vi "Log Write.vi"(6 "Controller Data In":refnum<data-value>, 7 "Write Header":bool, 8 "Measurement In":refnum<data-value>, 9 "State Estimate In":refnum<data-value>, 10 "Log Handle In":T1, 11 "Error In":errorcluster) -> (0 "Measurement Out":refnum<data-value>, 1 "State Estimate Out":refnum<data-value>, 2 "Log Handle Out":T1, 3 "Error Out":errorcluster, 4 "Controller Data Out":refnum<data-value>, 5 "Logged Events":string[](array[string]))   [LabVIEW 2021]
uses:
  State Estimator/Measurements.ctl
  IMU/IMU Data.ctl
  Steering Motor Encoder/Steering Motor Encoder Data.ctl
  GNSS/GNSS Data.ctl
  State Estimator/State Estimate.ctl
  Log Handle.ctl
  Controller Data.ctl
  Drive Motor/Drive Motor Data.ctl
  Steering Motor/Steering Motor Data.ctl
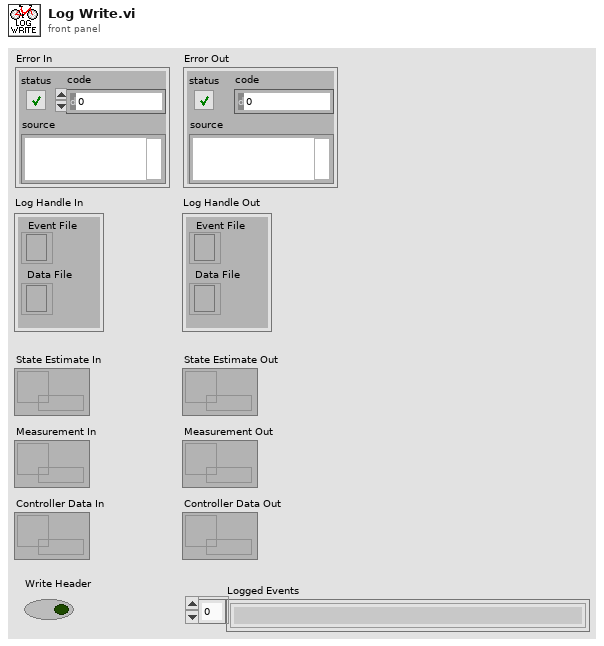
[diagram p1: front panel]
types:
  T1 = typedef "Log Handle.ctl" = cluster{"Data File":refnum<file>, "Event File":refnum<file>}
  T2 = typedef "State Estimate.ctl" = cluster{"X (m)":dbl, "Y (m)":dbl, "Psi (rad)":dbl, "Roll (rad)":dbl, "Roll Rate (rad/s)":dbl}
  T3 = typedef "Controller Data.ctl" = cluster{"Drive Motor Data":T4, "Steering Motor Data":T5}
  T4 = typedef "Drive Motor Data.ctl" = cluster{"Angular Speed (rad/s)":dbl, "Input Current (A)":dbl, "Motor Current (A)":dbl, "MOSFET Temperature (deg C)":dbl}
  T5 = typedef "Steering Motor Data.ctl" = cluster{"PWM":dbl, "Steering Angle Rate (rad/s)":dbl}
  T6 = typedef "Measurements.ctl" = cluster{"IMU Data":T7, "Steering Motor Encoder Data":T8, "GNSS Data":T9}
  T7 = typedef "IMU Data.ctl" = cluster{"Gyroscope":cluster{"X (rad/s)":dbl, "Y (rad/s)":dbl, "Z (rad/s)":dbl}, "Accelerometer":cluster{"X (m/s^2)":dbl, "Y (m/s^2)":dbl, "Z (m/s^2)":dbl}}
  T8 = typedef "Steering Motor Encoder Data.ctl" = cluster{"Encoder Position (counts)":i32, "Steering Angle (rad)":dbl}
  T9 = typedef "GNSS Data.ctl" = cluster{"Latitude (rad)":dbl, "Longitude (rad)":dbl, "Altitude (m)":dbl, "Speed (m/s)":dbl, "Heading (rad)":dbl, "Fix Quality":i32, "Number of Satellites":i32, "Latitude (deg)":dbl, "Longitude (deg)":dbl}
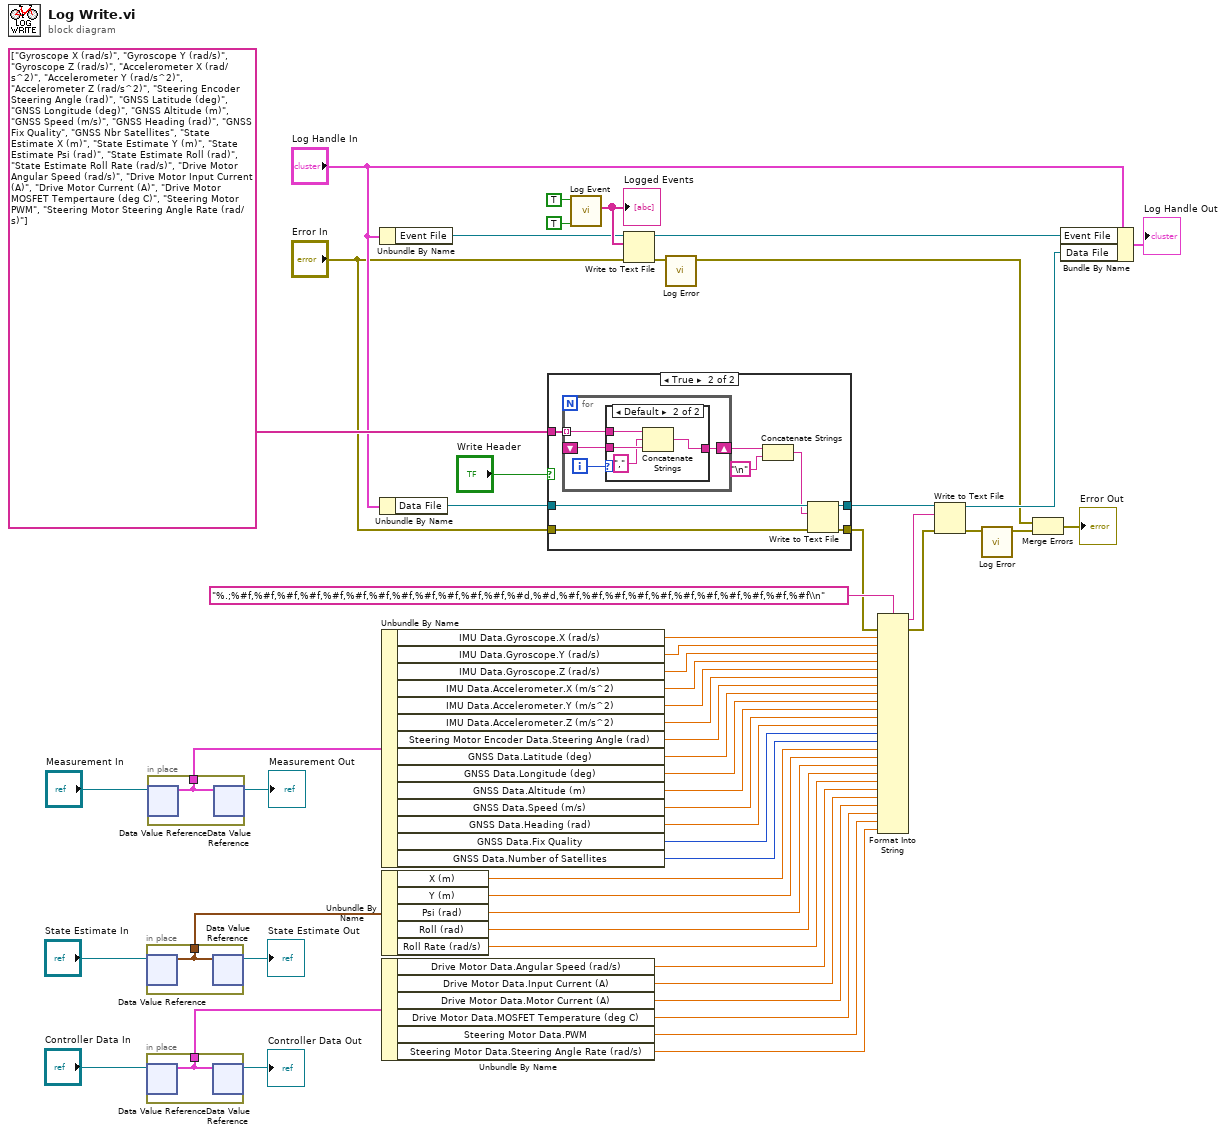
[diagram p0: block diagram]
diagram:
  n1 = in-place {
    in-place-border: [w57] -> w51
    n2 = in-place-dvr #1("State Estimate In") -> (w57:T2)  [unwired: 1 out]
    n3 = in-place-dvr #1(w57) -> (→"State Estimate Out":refnum<data-value>)  [unwired: 1 out]
  }
  n4 = in-place {
    in-place-border: [w58] -> w7
    n5 = in-place-dvr #2("Controller Data In") -> (w58:T3)  [unwired: 1 out]
    n6 = in-place-dvr #2(w58) -> (→"Controller Data Out":refnum<data-value>)  [unwired: 1 out]
  }
  n7 = in-place {
    in-place-border: [w59] -> w52
    n8 = in-place-dvr #3("Measurement In") -> (w59:T6)  [unwired: 1 out]
    n9 = in-place-dvr #3(w59) -> (→"Measurement Out":refnum<data-value>)  [unwired: 1 out]
  }
  n10 = Unbundle By Name("Log Handle In") -> ("Event File"=w19:refnum<file>)
  n11 = Unbundle By Name("Log Handle In") -> ("Data File"=w49:refnum<file>)
  n12 = Unbundle By Name(w52) -> ("IMU Data.Gyroscope.X (rad/s)"=w47:dbl, "IMU Data.Gyroscope.Y (rad/s)"=w46:dbl, "IMU Data.Gyroscope.Z (rad/s)"=w45:dbl, "IMU Data.Accelerometer.X (m/s^2)"=w44:dbl, "IMU Data.Accelerometer.Y (m/s^2)"=w43:dbl, "IMU Data.Accelerometer.Z (m/s^2)"=w42:dbl, "Steering Motor Encoder Data.Steering Angle (rad)"=w41:dbl, "GNSS Data.Latitude (deg)"=w40:dbl, "GNSS Data.Longitude (deg)"=w39:dbl, "GNSS Data.Altitude (m)"=w38:dbl, "GNSS Data.Speed (m/s)"=w37:dbl, "GNSS Data.Heading (rad)"=w36:dbl, "GNSS Data.Fix Quality"=w35:i32, "GNSS Data.Number of Satellites"=w34:i32)
  n13 = Unbundle By Name(w51) -> ("X (m)"=w32:dbl, "Y (m)"=w31:dbl, "Psi (rad)"=w30:dbl, "Roll (rad)"=w29:dbl, "Roll Rate (rad/s)"=w28:dbl)
  n14 = Unbundle By Name(w7) -> ("Drive Motor Data.Angular Speed (rad/s)"=w6:dbl, "Drive Motor Data.Input Current (A)"=w5:dbl, "Drive Motor Data.Motor Current (A)"=w4:dbl, "Drive Motor Data.MOSFET Temperature (deg C)"=w3:dbl, "Steering Motor Data.PWM"=w2:dbl, "Steering Motor Data.Steering Angle Rate (rad/s)"=w1:dbl)
  n15 = case shown="True" "Write Header" {
    tunnel: string[] ["Gyroscope X (rad/s)", "Gyroscope Y (rad/s)", "Gyroscope Z (rad/s)", "Accelerometer X (rad/s^2)", "Accelerometer Y (rad/s^2)", "Accelerometer Z (rad/s^2)", "Steering Encoder Steering Angle (rad)", "GNSS Latitude (deg)", "GNSS Longitude (deg)", "GNSS Altitude (m)", "GNSS Speed (m/s)", "GNSS Heading (rad)", "GNSS Fix Quality", "GNSS Nbr Satellites", "State Estimate X (m)", "State Estimate Y (m)", "State Estimate Psi (rad)", "State Estimate Roll (rad)", "State Estimate Roll Rate (rad/s)", "Drive Motor Angular Speed (rad/s)", "Drive Motor Input Current (A)", "Drive Motor Current (A)", "Drive Motor MOSFET Tempertaure (deg C)", "Steering Motor PWM", "Steering Motor Steering Angle Rate (rad/s)"] ("channel name(s) in (Untitled)") -> [_ w69]
    tunnel: w49 -> [w61 w68]
    tunnel: "Error In" -> [w60 w67]
    tunnel: [w61 w66] -> w27
    tunnel: [w60 w65] -> w25
    frame False {
    }
    frame True {
      n16 = for {
        tunnel: w69 -> [w73] mode=indexing
        shift-right: [w71] -> w64
        shift-left: _ -> [w70]
        i -> [w72]
        n17 = case shown="Default" w72 {
          tunnel: w73 -> [w74 w78]
          tunnel: [w74 w77] -> w71
          tunnel: w70 -> [_ w76]
          frame 0 {
          }
          frame Default {
            n18 = Concatenate Strings(w78, "," ("string"), w76) -> (w77:string)
          }
        }
      }
      n19 = Concatenate Strings(w64, "\n") -> (w63:string)
      n20 = Write to Text File(file (use dialog)=w68, text=w63, error in=w67) -> (refnum out=w66:refnum<file>, error out=w65:errorcluster)  [unwired: 1 in, 1 out]
    }
  }
  n21 = call "Log Event.vi"("Clear Log"=TRUE, "Read"=TRUE) -> ("All Events"=w21:string[])  [unwired: 9 in]
  "Logged Events" <- w21
  n22 = Write to Text File(file (use dialog)=w19, text=w21, error in="Error In") -> (refnum out=w16:refnum<file>, error out=w15:errorcluster)  [unwired: 1 in, 1 out]
  n23 = call "Log Error.vi"("Error In"=w15) -> ("Error Out"=w12:errorcluster)  [unwired: 10 in]
  n24 = Format Into String(format string="%.;%#f,%#f,%#f,%#f,%#f,%#f,%#f,%#f,%#f,%#f,%#f,%#f,%#d,%#d,%#f,%#f,%#f,%#f,%#f,%#f,%#f,%#f,%#f,%#f,%#f\\n", error in=w25, w47, w46, w45, w44, w43, w42, w41, w40, w39, w38, w37, w36, w35, w34, w32, w31, w30, w29, w28, w6, w5, w4, w3, w2, w1) -> (resulting string=w26:string, error out=w24:errorcluster)  [unwired: 1 in]
  n25 = Write to Text File(file (use dialog)=w27, text=w26, error in=w24) -> (refnum out=w17:refnum<file>, error out=w14:errorcluster)  [unwired: 1 in, 1 out]
  n26 = call "Log Error.vi"("Error In"=w14) -> ("Error Out"=w13:errorcluster)  [unwired: 10 in]
  n27 = Merge Errors(w12, w13) -> (→"Error Out":errorcluster)
  n28 = Bundle By Name(cluster="Log Handle In", "Event File"=w16, "Data File"=w17) -> (→"Log Handle Out":T1)
